vi "Security System Demo.vi"() -> ()   [LabVIEW 2014]
uses:
  Security System/Security Level.ctl
  Door Alarm/Door Alarm.lvclass
  Motion Detectors/Motion Detectors.lvclass
  Threat Deterent/Threat Deterent.lvclass
  Security System/Security System.lvclass
panel:
  out "Last Action Performed":string
  in  "stop":bool
  in  "Security Level":T1
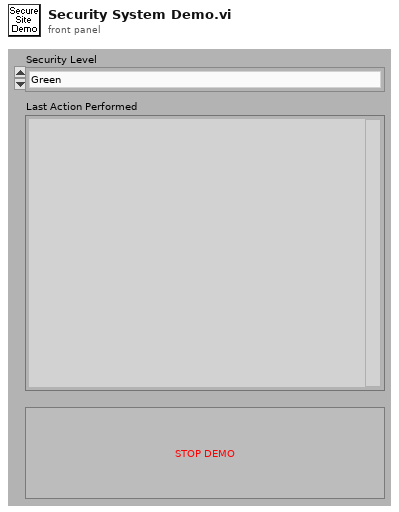
[diagram p1: front panel]
types:
  T1 = typedef "Security System.lvclass/Security Level.ctl" = enum16{"Green", "Yellow", "Orange", "Red"}
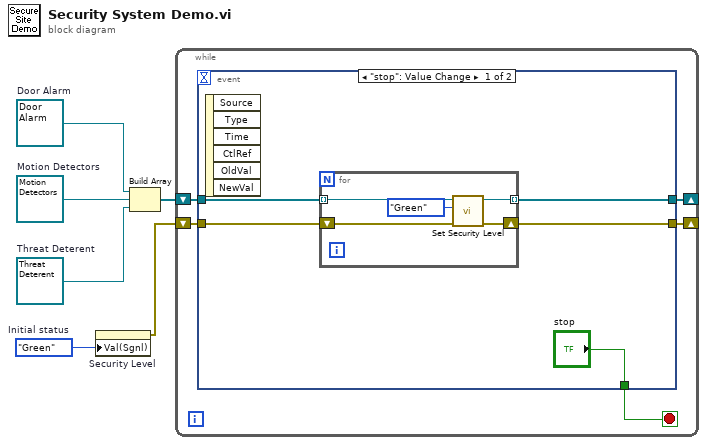
[diagram p0: block diagram]
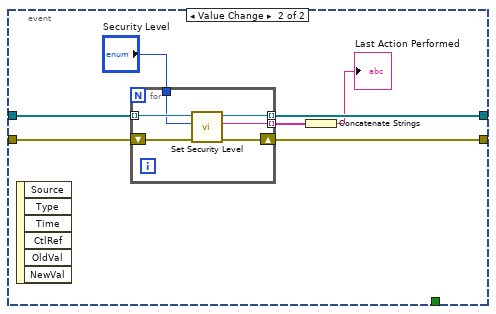
[diagram p2: hidden frame]
diagram:
  w2 = enum16{"Green", "Yellow", "Orange", "Red"}."Green"  # Initial status
  w4 = refnum<class "Threat Deterent.lvclass"> refnum  # Threat Deterent
  w5 = refnum<class "Motion Detectors.lvclass"> refnum  # Motion Detectors
  w6 = refnum<class "Door Alarm.lvclass"> refnum  # Door Alarm
  n1 = property on="Security Level" class="Enum (strict)"("Val(Sgnl)"=w2) -> (error out=w1:errorcluster)  [unwired: 2 in, 1 out]
  n2 = Build Array(w6, w5, w4) -> (w3:refnum<class "Security System.lvclass">[])
  n3 = while {
    shift-right: [w10] -> _
    shift-left: w3 -> [w9]
    shift-right: [w8] -> _
    shift-left: w1 -> [w7]
    stop <- w11 stop-if-true
    n4 = event shown="[0] \"stop\": Value Change" {
      selector: _ -> [_ _]
      dyn-events: _ -> [_ _]
      timeout: _ -> [_ _]
      tunnel: ["stop" _] -> w11
      tunnel: [w14 w27] -> w10
      tunnel: w9 -> [w15 w28]
      tunnel: [w13 w26] -> w8
      tunnel: w7 -> [w12 w25]
      event "stop": Value Change {
        n5 = event-data() -> ()  [unwired: 1 in, 6 out]
        n6 = for {
          tunnel: w15 -> [w21] mode=indexing
          tunnel: [w20] -> w14 mode=indexing
          shift-right: [w18] -> w13
          shift-left: w12 -> [w17]
          n7 = call "Set Security Level.vi"("error in (no error)"=w17, "New Level"=Security_Level."Green", "Security System in"=w21) -> ("error out"=w18:errorcluster, "Security System out"=w20:refnum<class "Security System.lvclass">)  [unwired: 6 in, 1 out]
        }
      }
      event Value Change {
        n8 = event-data() -> ()  [unwired: 1 in, 6 out]
        n9 = for {
          tunnel: w28 -> [w34] mode=indexing
          tunnel: [w33] -> w27 mode=indexing
          shift-right: [w32] -> w26
          shift-left: w25 -> [w31]
          tunnel: "Security Level" -> [w30]
          tunnel: [w29] -> w23 mode=indexing
          n10 = call "Set Security Level.vi"("error in (no error)"=w31, "New Level"=w30, "Security System in"=w34) -> ("error out"=w32:errorcluster, "Last Action Performed"=w29:string, "Security System out"=w33:refnum<class "Security System.lvclass">)  [unwired: 6 in]
        }
        n11 = Concatenate Strings(w23) -> (→"Last Action Performed":string)
      }
    }
  }
